vi "Main_06B.vi"() -> ()   [LabVIEW 2024]
uses:
  ENUM_Direction.ctl
panel:
  out "It":i32
  out "count":i32
  out "2D Array":string[][](array[string])
  in  "Select Puzzle":bool
  out "Answer":u32
  in  "Puzzle":string="..........#...........#...........#.............................#......................#.........#................................\n..........................#.........#......#.................................#...........................#........................\n..................................#...#................................................................................#..........\n.#...............#.....#..........#.........#......#........#................................#......#.............................\n...#.......#.............#.............................................#.........##...............#.................#.............\n.......................................#.............#..................#........#.......#.........#...............#.........#....\n.....#..................#..#..#.........................#...................#....#........#.............................#.........\n.......#.............................#..........#......#..........................##......#.......................##..............\n.....#.....#........................................................................................#.......#.....................\n.................................#............#...#.....................................................#.........#...............\n...............#.....#..#....#....#.....................................................#............#........#.#.................\n.......#.....#...........................................................#............................#.................#....#....\n...........................#.................#....................................#...............#..#........................#...\n.....#.........................................#.................#...##....................................#......................\n.............#...#..................#......#.................#..........................................#.....#..........#........\n.................#...............#............#.......#.#...............................................#..................#......\n.....#..#.....................#.......................................................#..............#..............#.......##....\n..##........#....................................................#.............#..............#........................#..#.......\n..............................#...........#...#........................#............#..........................#........#........#\n.....................................##...............................#............#............#....#............................\n...##........................#.....#....#.........#.................................................#.............................\n...............................#................................#...............#.....#.....................#.....................\n................................................#..........#....#............................#.....#.......#..................#...\n.............#.....#.........#.#....#................##......#.............#......................................................\n..........#..............#..........#......#.........#...#.........................................#.#.....#.........#............\n..................#......................#.............................#...................#.....................................#\n................#.....#..............................#.............#.............#..#.....#....................................#..\n.........#.#................#.........#.................#...................#................................#................#...\n.............................................................#..............#.....................................................\n......#.........................#...........#.........#..................#....................................#..#...........##...\n.............................................................................#.............#........................#...#.........\n......#......#..#............#..............................................#....#..#..#................#.........#....#..........\n........#........#.........#....................................................^..#...#....................#...............#.....\n..#....#...#.......................................................................................................#..............\n.....#...........................................#..............#.........#....#........................................#.........\n.....................................#..............#............................................................#................\n.....#.......................#........................#..........#.............#.................#..................#.............\n.......................................#......#.....................................#.........................#...................\n...........................................................................................#............................##........\n..#............#..........................#...........#...#..................#......#.................#.#.................#......#\n.###......#....................#...#...........................................................#.........#.....#..............#.#.\n....................................#..........#.....#.......................#...............#.....#......#...................#...\n...#......#..................#......#.......#..............#..............#.......................................................\n..........#....................................................................#................##.#...#..........................\n.........................................................#..................##.....................#..##..........................\n..................#......#.................................#.................#.##................................................#\n...#..........#...#..#..............................................#...........................##........#.......................\n.....#................................................#...........#..................#...#.................................#......\n.......#.....#.........................#..........................................................................................\n....................................................#........#....#....................................##..............#.....#....\n............#........#.........................#.................................#..........................................#...#.\n.....................................#........................#...................#......#.#...........#..#..........#...........#\n................#...............#.........................#.........................#........#..#.................................\n.............#.........#.............#.#.#.........#...................#.......#.......................#..........................\n.............#......................................................#................................................#.......#....\n....#....................................................................#.#........#.................#..........................#\n.................................#......#....................................................................#.....#..............\n............##...................#.......................................................................#.........#........#.....\n#..................................................#..#...............#............#.............#...............................#\n.............................#.................................#.....#..........................#.............#..#...#...#........\n...#.....#..............................#.#......................................#................................................\n...#............##...............................#............#..............................#................................#...\n#.................#......##..............................................................#...........#........#...#...............\n....##.....................................................................................................#.#....................\n#.................#..................................................#..................................................#.........\n.........#.........#...........................#.................#.#.............................#................................\n................................#............#................................................................#...................\n.....................................#............................................#.##......##........#...........................\n....#....................................................#...#.#.#....................................................#...........\n.........................#.#...................#...................##...............#........................#....................\n..................................#...................................................................#.......#..................#\n...................#.............................................#.......................#.#.....................#....#...........\n#....................................#.#..#.#..........#.........#.........##.........#......................#............#.......\n...............................................................#.............................##....#.......#......................\n.............#......#.#.........#............................#............................#.......................................\n......................#.........#.........................................................#...#............#......................\n...................#.....#.....................................................#.....................................#............\n...............................#.....#..................#.......##................................................................\n.............................................#.........................#...........#..............................#..#............\n#..##..................................................................................................#......#...........#.....#.\n.......................................................#.....................#.............................#......................\n...........................................................................................................#......................\n......................#..............................................................#............................................\n...........................#.....#......................................#.........#........#..#.#.................................\n.#.......#........................................................................................................................\n.#.......#...........................................#................................#...........................................\n.........................................................#........................................#......#........................\n...............................#...#........#............................................#.................#......................\n......#.........................#......................#.....#.#..............#..................#.......#..................#.....\n.................#........#...#........................#.............................#............................................\n#...........................................................................#............................#................#.......\n..........................................................................#................#......................................\n.............#.............................................................................#.........................#............\n.#...........#.......#.......#.....#....#.......#........#....................#........................#........................#.\n...#..............#.............................#.............................................................#...#..#..........#.\n......#......#.#...............##................................................................................................#\n....#........#.##......#...#......................................................................................................\n..#..#.#.#.....................#................................#...................................#.....#...#...................\n.....................#.#........#..............##..............#.................#..............................................#.\n...................................................................................#........#.......#....#............#...........\n.....#....#..................#...............#.............................................#.#....................#...............\n.....................#..........#............#..................................#......................#.#.....#................#.\n..........#.........................................#...............#.............................................................\n.......#......................#.............#.....#..............#........................#.....#.........#.................#...#.\n..................................................................#.....#...............................................#........#\n.......#..........#.......#....#.......#..........#....#............................................#.#...........................\n..#...........#..............................#....................#....................#...#......................................\n.......#...............................#............#.....#.....................#.................................................\n.........#..................#..................#..................................................................................\n..........................................................................................#....#...................#.......##.....\n..................#.............................##.......................................................#.......#......#......#..\n...#.......#..............................................................................................#.......................\n............#..#..............................................................#...........##....#....#.#................#........#\n............#.........................#........#....#..#..................................#..................#....................\n......##......................#...##..............................#...............................................................\n........................#................#..............#...##...............................#..................##....#...........\n....#.#...#.....#..................................#..............................#...........#.....................#.............\n......................#.........................................................................#..........#.............#........\n.#......#............................................................#...............................#...#........................\n.......##.....................#.....#...........#......##.......##...................#...............................#............\n...#...#........#...............#......#......#.....#...#.................................................................#.......\n..................#.......................#...............................................#.................#.............#..#....\n.....................#.......#....#...#............................#.....................#............#.....................#.....\n................................................................#....#......#............#..................#.........#...........\n.......................#...................#..............................................................................###.....\n...............................#...........#................................#........#..#....#............................#.......\n....#......#...............................#...............#......................................#...............................\n...........#...........................##.........................................................................#.#.............\n.........................#.........#.........................................#.....#...................#.....#.......#............\n.............................#.....#................##..#.....................#..................................................."
  in  "Example":string="....#.....\n.........#\n..........\n..#.......\n.......#..\n..........\n.#..^.....\n........#.\n#.........\n......#..."
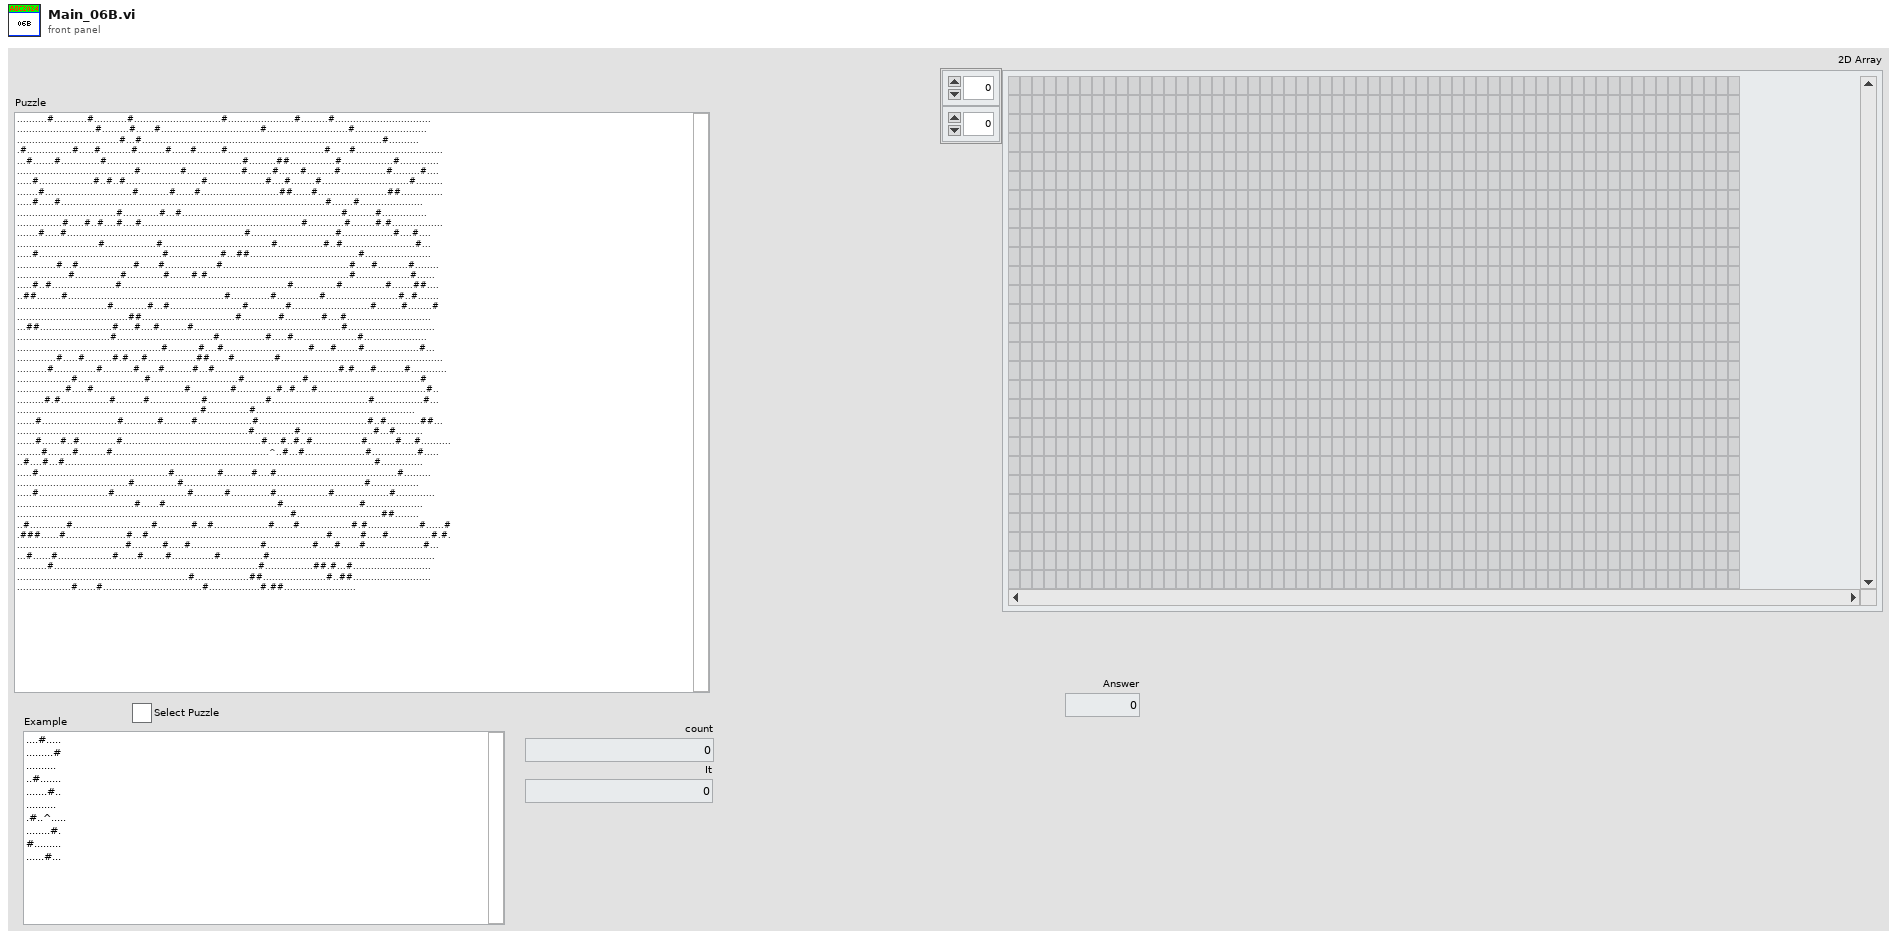
[diagram p1: front panel]
types:
  T1 = typedef "ENUM_Direction.ctl" = enum16{"Up;-1,0", "Right;0,1", "Down;1,0", "Left;0,-1"}
  T2 = set{cluster{"Direction":T1, "Position":cluster{i32, "index of element":i32}}}
  T3 = cluster{"Direction":T1, cluster{i32, "index of element":i32}}
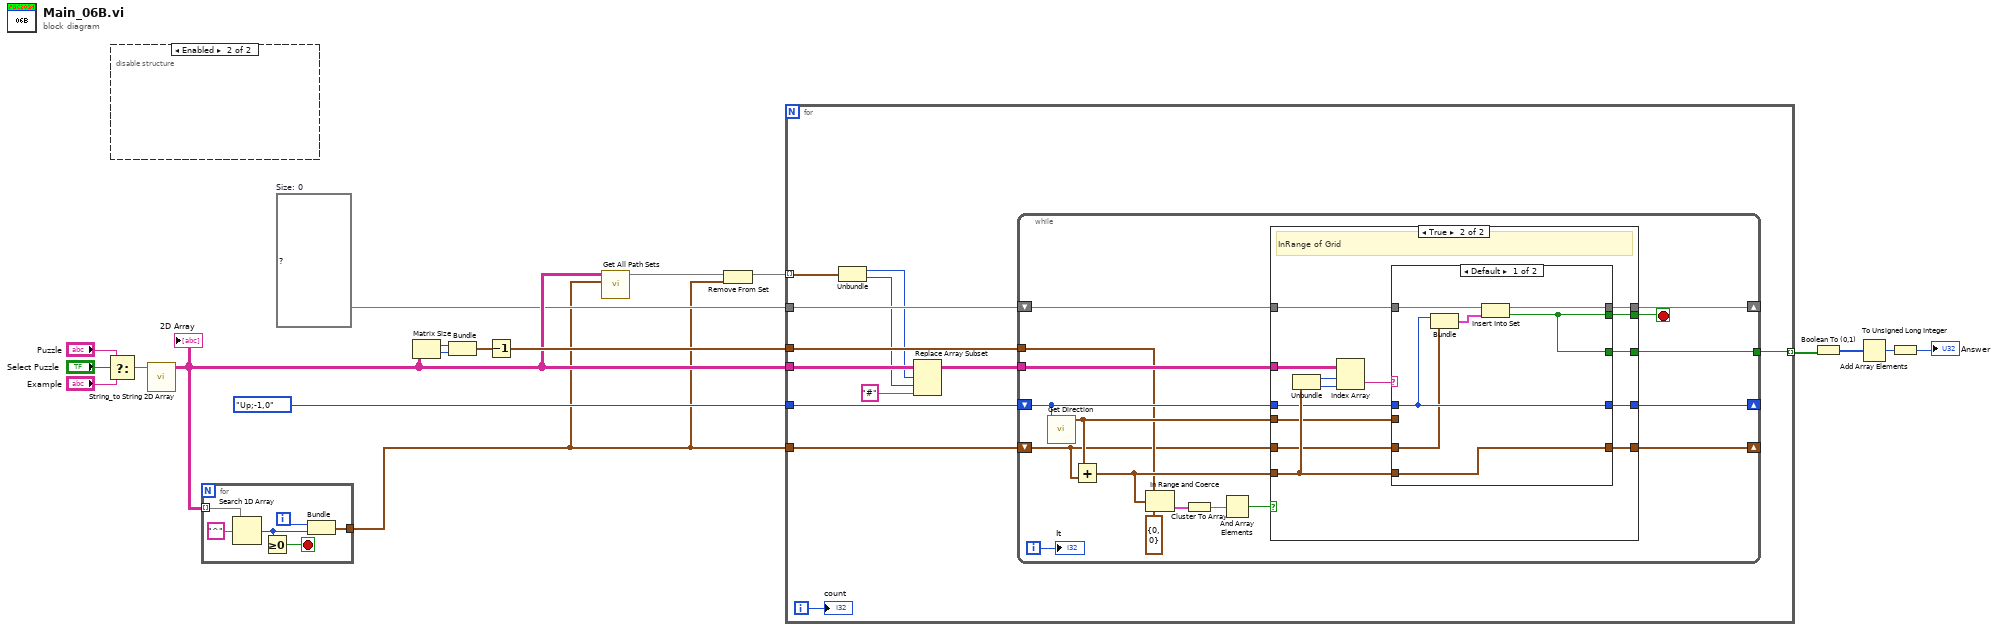
[diagram p0: block diagram]
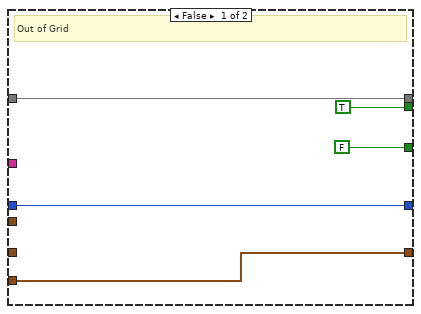
[diagram p2: hidden frame]
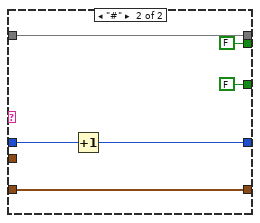
[diagram p3: hidden frame]
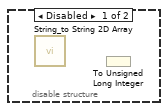
[diagram p4: hidden frame]
diagram:
  w3 = T2 {}  # Size: 0
  n1 = Select(t="Puzzle", s="Select Puzzle", f="Example") -> (s? t:f=w15:string)
  n2 = disable-structure shown="Enabled" {
    frame Disabled {
      n3 = call "String_to String 2D Array.vi"() -> ()  [unwired: 11 in, 1 out]
      n4 = To Unsigned Long Integer() -> ()  [unwired: 1 in, 1 out]
    }
    frame Enabled {
    }
  }
  n5 = call "String_to String 2D Array.vi"("Input String"=w15) -> ("2D Array"=w9:string[][])  [unwired: 10 in]
  "2D Array" <- w9
  n6 = for {
    tunnel: w9 -> [w24] mode=indexing
    tunnel: [w19] -> w2
    i -> [w21]
    stop <- w22 stop-if-true
    n7 = Search 1D Array(1D array=w24, element="^") -> (index of element=w20:i32)  [unwired: 1 in]
    n8 = Greater Or Equal To 0?(x=w20) -> (x >= 0?=w22:bool)
    n9 = Bundle(w21, "index of element"=w20) -> (w19:cluster{i32, "index of element":i32})  [unwired: 1 in]
  }
  n10 = Matrix Size(0:w9) -> (1:w14:i32, 2:w13:i32)
  n11 = Bundle("number of columns"=w14, "matrix"=w13) -> (w12:cluster{"number of columns":i32, "matrix":i32})  [unwired: 1 in]
  n12 = Decrement(x=w12) -> (x-1=w10:cluster{"number of columns":i32, "matrix":i32})
  n13 = call "Get All Path Sets.vi"("Start"=w2, "2D Array"=w9) -> ("Set"=w8:set{cluster{i32, "index of element":i32}})  [unwired: 9 in]
  n14 = Remove From Set(10:w2, 11:w8) -> (3:w1:set{cluster{i32, "index of element":i32}})  [unwired: 1 out]
  n15 = for {
    tunnel: w3 -> [w36]
    tunnel: w9 -> [w35]
    tunnel: ENUM_Direction."Up;-1,0" ("Direction") -> [w34]
    tunnel: w2 -> [w33]
    tunnel: w10 -> [w32]
    tunnel: w1 -> [w31] mode=indexing
    tunnel: [w26] -> w7 mode=indexing
    i -> [w25]
    n16 = Unbundle(w31) -> (w29:i32, "index of element"=w28:i32)
    n17 = Replace Array Subset(array=w35, new element="#" ("new element/subarray"), index (row)=w29, index (col)=w28) -> (w30:string[][])
    n18 = while {
      tunnel: w30 -> [w53]
      shift-right: [w49] -> _
      shift-left: w33 -> [w42]
      shift-right: [w47] -> _
      shift-left: w34 -> [w48]
      shift-right: [w51] -> _
      shift-left: w36 -> [w52]
      tunnel: w32 -> [w45]
      tunnel: [w41] -> w26
      i -> [w37]
      stop <- w43 stop-if-true
      n19 = call "Get Direction.vi"("Direction"=w48) -> ("Direction"=w50:cluster{"Numeric":i32, "Numeric":i32})  [unwired: 10 in]
      n20 = Add(x=w50, y=w42) -> (x+y=w46:cluster{i32, i32})
      n21 = In Range and Coerce(upper limit=w45, x=w46, lower limit=cluster{"number of columns":i32, "matrix":i32} {"number of columns"=0, "matrix"=0}) -> (In Range?=w40:cluster{"number of columns":bool, "matrix":bool})  [unwired: 1 out]
      n22 = Cluster To Array(cluster=w40) -> (array=w39:bool[])
      n23 = And Array Elements(Boolean array=w39) -> (logical AND=w38:bool)
      n24 = case shown="True" w38 {
        tunnel: w53 -> [_ w72]
        tunnel: w52 -> [w58 w68]
        tunnel: [w58 w67] -> w51
        tunnel: w46 -> [w56 w66]
        tunnel: w50 -> [_ w59]
        tunnel: [w56 w65] -> w49
        tunnel: w48 -> [w57 w64]
        tunnel: [w57 w63] -> w47
        tunnel: [TRUE w61] -> w43
        tunnel: w42 -> [_ w62]
        tunnel: [FALSE ("already included?") w60] -> w41
        frame False {
          # "Out of Grid"
        }
        frame True {
          # "InRange of Grid"
          n25 = Unbundle(w66) -> (w71:i32, w70:i32)
          n26 = Index Array(array=w72, index (row)=w71, index (col)=w70) -> (element=w69:string)
          n27 = case shown="Default" w69 {
            tunnel: w68 -> [w79 w85]
            tunnel: [w78 w85] -> w67
            tunnel: w66 -> [w74 _]
            tunnel: [w74 w82] -> w65
            tunnel: w64 -> [w77 w84]
            tunnel: [w77 w83] -> w63
            tunnel: w62 -> [w73 w82]
            tunnel: [w75 FALSE ("already included?")] -> w61
            tunnel: [w75 FALSE ("already included?")] -> w60
            tunnel: w59 -> [_ _]
            frame Default {
              n28 = Bundle("Direction"=w77, w73) -> (w76:T3)  [unwired: 1 in]
              n29 = Insert Into Set(10:w76, 11:w79) -> (2:w75:bool, 3:w78:T2)
            }
            frame "#" {
              n30 = Increment(x=w84) -> (x+1=w83:T1)
            }
          }
        }
      }
      "It" <- w37
    }
    "count" <- w25
  }
  n31 = Boolean To (0,1)(Boolean=w7) -> (0, 1=w6:i16[])
  n32 = Add Array Elements(numeric array=w6) -> (sum=w5:i16)
  n33 = To Unsigned Long Integer(number=w5) -> (unsigned 32bit integer=→"Answer":u32)
